vi "Global Data!!!.vi"() -> ()   [LabVIEW 2014]
panel:
  in  "straightDrive":bool
  in  "Turn":dbl
  in  "Power":dbl
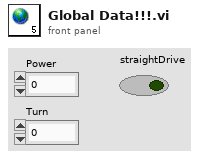
[diagram p1: front panel]
diagram:
